vi "power PID.vi"(6 "nonzero temperature":dbl=300.0, 7 "control power PID?":bool, 10 "sweep folder path":path, 11 "Fast sweep settings":T1={"Update rate (Hz)"=250.0, "Start F, Hz"=300000.0, "Stop F"=3500000.0, "Number of points"=23000, "Amplitude"=0.2, "Init&amplitude"=TRUE, "IF"=1000.0, "Time constant"=0.001} {"IF" format="%#_6p"; "Amplitude" min=0.0 max=2.5; "Number of points" format="%.0p"; "Stop F" format="%#_6p"; "Start F, Hz" format="%#_6p"; "Update rate (Hz)" format="%0.2f"}) -> (3 "Fast sweep settings out":T1={"Update rate (Hz)"=250.0, "Start F, Hz"=200000.0, "Stop F"=1700000.0, "Number of points"=30000, "Amplitude"=2.1, "Init&amplitude"=TRUE, "IF"=1000.0, "Time constant"=0.1} {"IF" format="%#_6p"; "Amplitude" min=0.0 max=2.5; "Number of points" format="%.0p"; "Stop F" format="%#_6p"; "Start F, Hz" format="%#_6p"; "Update rate (Hz)" format="%0.2f"})   [LabVIEW 2010]
uses:
  RUS/Controls/Sweep settings.ctl
  next chunk read-write PID -- action.ctl
  array -- find index - real.vi
  Q - not nan -- real.vi
  file -- read list of lines.vi
  parse -- find first line.vi
  parse -- get list of matches -- numbers.vi
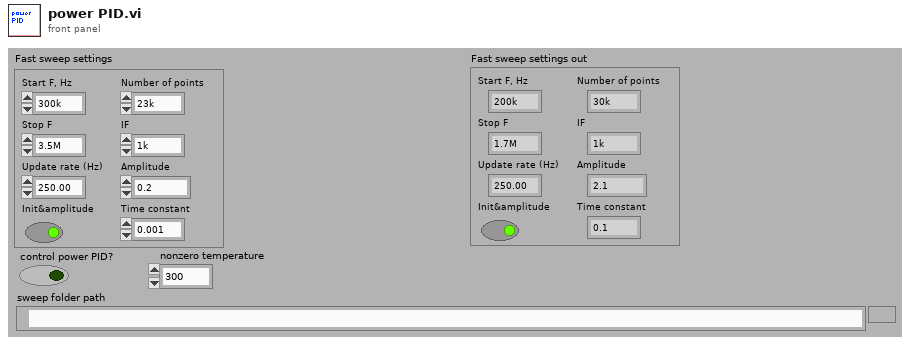
[diagram p1: front panel]
types:
  T1 = typedef "Sweep settings.ctl" = cluster{"Update rate (Hz)":dbl, "Start F, Hz":dbl, "Stop F":dbl, "Number of points":i32, "Amplitude":dbl, "Init&amplitude":bool, "IF":dbl, "Time constant":dbl}
  T2 = typedef "next chunk read-write PID -- action.ctl" = enum16{"read", "interpolate", "append col", "write", "write PID col", "append PID col"}
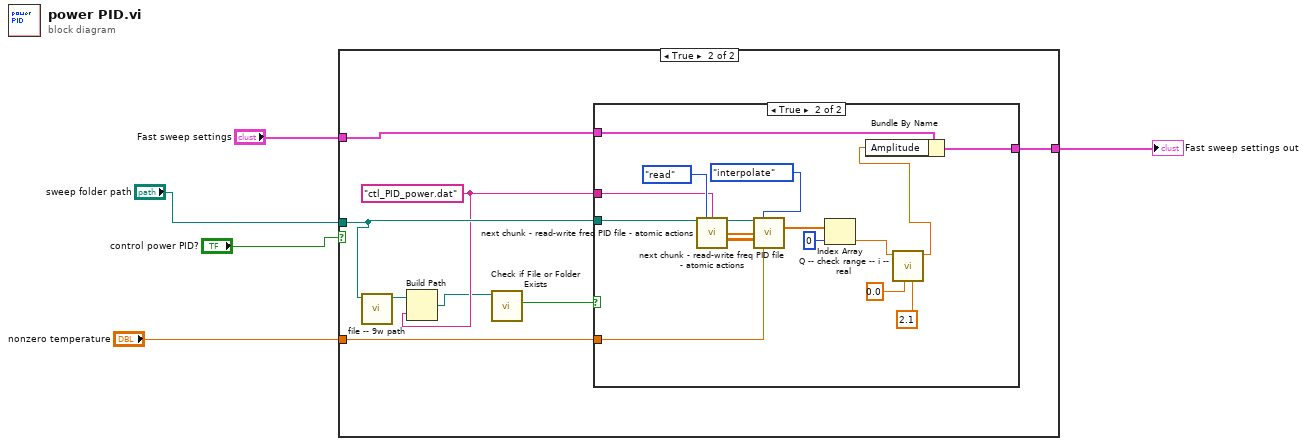
[diagram p0: block diagram]
diagram:
  n1 = case shown="True" "control power PID?" {
    tunnel: "Fast sweep settings" -> [w6 w8]
    tunnel: "sweep folder path" -> [_ w13]
    tunnel: "nonzero temperature" -> [_ w9]
    tunnel: [w6 w7] -> w1
    frame False {
    }
    frame True {
      w12 = "ctl_PID_power.dat" ("freq PID file OUT")
      n2 = call "file -- 9w path.vi"("sweep folder"=w13) -> ("9w path"=w14:path)  [unwired: 10 in]
      n3 = Build Path(base path=w14, name or relative path=w12) -> (appended path=w11:path)
      n4 = call <vilib>:"Check if File or Folder Exists.vi"("path"=w11) -> ("file or folder exists?"=w10:bool)  [unwired: 8 in, 2 out]
      n5 = case shown="True" w10 {
        tunnel: w13 -> [_ w28]
        tunnel: w12 -> [_ w20]
        tunnel: w9 -> [_ w27]
        tunnel: w8 -> [w15 w24]
        tunnel: [w15 w23] -> w7
        frame False {
        }
        frame True {
          n6 = call "next chunk - read-write freq PID file - atomic actions .vi"("sweep folder path"=w28, "PID action"=next_chunk_read-write_PID_--_action."read", "freq PID file IN"=w20) -> ("sweep folder path out"=w30:path, "temperatures"=w21:dbl[], "frequencies"=w22:dbl[][])  [unwired: 8 in, 2 out]
          n7 = call "next chunk - read-write freq PID file - atomic actions .vi"("sweep folder path"=w30, "PID action"=next_chunk_read-write_PID_--_action."interpolate", "temperatures IN"=w21, "frequencies IN"=w22, "temperature"=w27) -> ("PID freq"=w26:dbl[])  [unwired: 6 in, 4 out]
          n8 = Index Array(array=w26, index=0) -> (element=w19:dbl)
          n9 = call "Q -- check range -- i -- real.vi"("upper"=2.1, "lower"=0.0, "number"=w19) -> ("number in range"=w17:dbl)  [unwired: 6 in, 2 out]
          n10 = Bundle By Name(cluster=w24, "Amplitude"=w17) -> (w23:T1)
        }
      }
    }
  }
  "Fast sweep settings out" <- w1
